vi "my Write Controls on Tab to Config File.vi"(4 "error in":errorcluster, 6 "Page Refnum":refnum<vi>, 7 "configuration file path":path) -> (0 "error out":errorcluster, 3 "configuration file path out":path)   [LabVIEW 2019]
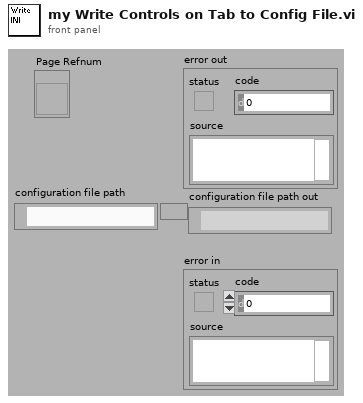
[diagram p1: front panel]
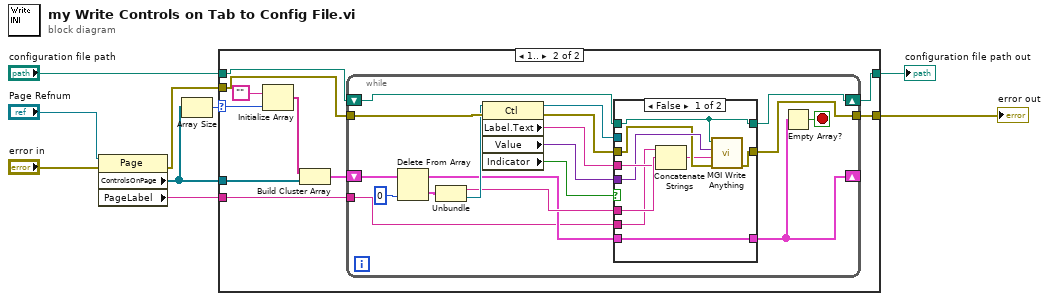
[diagram p0: block diagram]
diagram:
  n1 = property class="Page"(reference="Page Refnum", error in="error in") -> (error out=w7:errorcluster, "ControlsOnPage"=w5:refnum<vi>[], "PageLabel"=w4:string)  [unwired: 1 out]
  n2 = Array Size(array=w5) -> (size(s)=w3:i32)
  n3 = case shown="1.." w3 {
    selector: w3 -> [_ w12]
    tunnel: w7 -> [w11 w21]
    tunnel: "configuration file path" -> [w10 w20]
    tunnel: [w11 w19] -> w6
    tunnel: [w10 w18] -> w2
    tunnel: w5 -> [_ w15]
    tunnel: w4 -> [_ w13]
    frame 0, Default {
    }
    frame 1.. {
      n4 = Initialize Array("", w12) -> (w16:string[])
      n5 = Build Cluster Array(w16, w15) -> (w14:cluster{string, refnum<vi>}[])
      n6 = while {
        shift-right: [w37] -> w18
        shift-left: w20 -> [w38]
        tunnel: w21 -> [w36]
        tunnel: [w34] -> w19
        shift-right: [w24] -> _
        shift-left: w14 -> [w32]
        tunnel: w13 -> [w23]
        stop <- w27 stop-if-true
        n7 = Delete From Array(array=w32, index=0) -> (deleted portion=w33:cluster{string, refnum<vi>}, array with subset deleted=w26:cluster{string, refnum<vi>}[])  [unwired: 1 in]
        n8 = Unbundle(w33) -> (w29:string, w30:refnum<vi>)
        n9 = property class="Ctl"(reference=w30, error in=w36) -> (reference out=w25:refnum<vi>, error out=w35:errorcluster, "Label.Text"=w28:string, "Value"=w39:variant, "Indicator"=w22:bool)
        n10 = case shown="False" w22 {
          tunnel: w39 -> [w46 _]
          tunnel: w38 -> [w42 w51]
          tunnel: [w42 w51] -> w37
          tunnel: w35 -> [w44 w50]
          tunnel: [w43 w50] -> w34
          tunnel: w29 -> [w48 _]
          tunnel: w28 -> [w47 _]
          tunnel: w26 -> [w45 w49]
          tunnel: w25 -> [_ _]
          tunnel: [w45 w49] -> w24
          tunnel: w23 -> [w41 _]
          frame False {
            n11 = Concatenate Strings(w41, w48, w47) -> (w40:string)
            n12 = call <userlib>:"MGI Write Anything.vi"("Error In"=w44, "Section Name (Name of \"Anything\")"=w40, "Anything"=w46, "Path (dialog)"=w42) -> ("Error Out"=w43:errorcluster)  [unwired: 5 in, 2 out]
          }
          frame True {
          }
        }
        n13 = Empty Array?(array=w24) -> (empty?=w27:bool)
      }
    }
  }
  "error out" <- w6
  "configuration file path out" <- w2
